vi "specu1a 1.0.0 Find Spectrometer by name.vi"(3 "All Spectrometers":T1[](array[typedef]) {"White"."Spectrum" format="%.2f"; "Data"."Spectrum" format="%.2f"; "Dark"."Spectrum" format="%.2f"}, 5 "Name":string) -> (0 "All Spectrometers out":T1[](array[typedef]) {"White"."Spectrum" format="%.2f"; "Data"."Spectrum" format="%.2f"; "Dark"."Spectrum" format="%.2f"}, 1 "Single Spectrometer":T1={"USB"={"pUSB"=0, "Pipe"=0, "No of Avgs"=0, "SYS Number"="", "DLL Number"=""}, "Unit Information"={"UnitID"="", "Sensor Name"="", "Serial Number"="", "Reserved"="", "Wave Upper"=630, "Wave Lower"=1050}, "Dark"={"Spectrum"=[], "Parameters"={"Integration time"=0, "Gain"=enum."Low", "TriggerEdge"=enum."Rising", "Trigger Mode"=enum."Internal", "Reserved"=0}, "No of Avgs"=0}, "Data"={"Spectrum"=[], "Parameters"={"Integration time"=0, "Gain"=enum."Low", "TriggerEdge"=enum."Rising", "Trigger Mode"=enum."Internal", "Reserved"=0}, "No of Avgs"=0}, "White"={"Spectrum"=[], "Parameters"={"Integration time"=10000, "Gain"=enum."Low", "TriggerEdge"=enum."Rising", "Trigger Mode"=enum."Internal", "Reserved"=0}, "No of Avgs"=0}, "Parameters"={"Integration time"=10000, "Gain"=enum."Low", "TriggerEdge"=enum."Rising", "Trigger Mode"=enum."Internal", "Reserved"=0}} {"White"."Spectrum" format="%.2f"; "Data"."Spectrum" format="%.2f"; "Dark"."Spectrum" format="%.2f"}, 2 "index of element":i32)   [LabVIEW 2010]
uses:
  Controls/specu1a 1.0.0 Single spectrometer.ctl
  Controls/specu1a 1.0.0 Product Information.ctl
  Controls/specu1a 1.0.0 Single measurement.ctl
  Controls/specu1a 1.0.0 Parameters.ctl
  Controls/specu1a 1.0.0 Trigger Edge.ctl
  Controls/specu1a 1.0.0 Trigger Mode.ctl
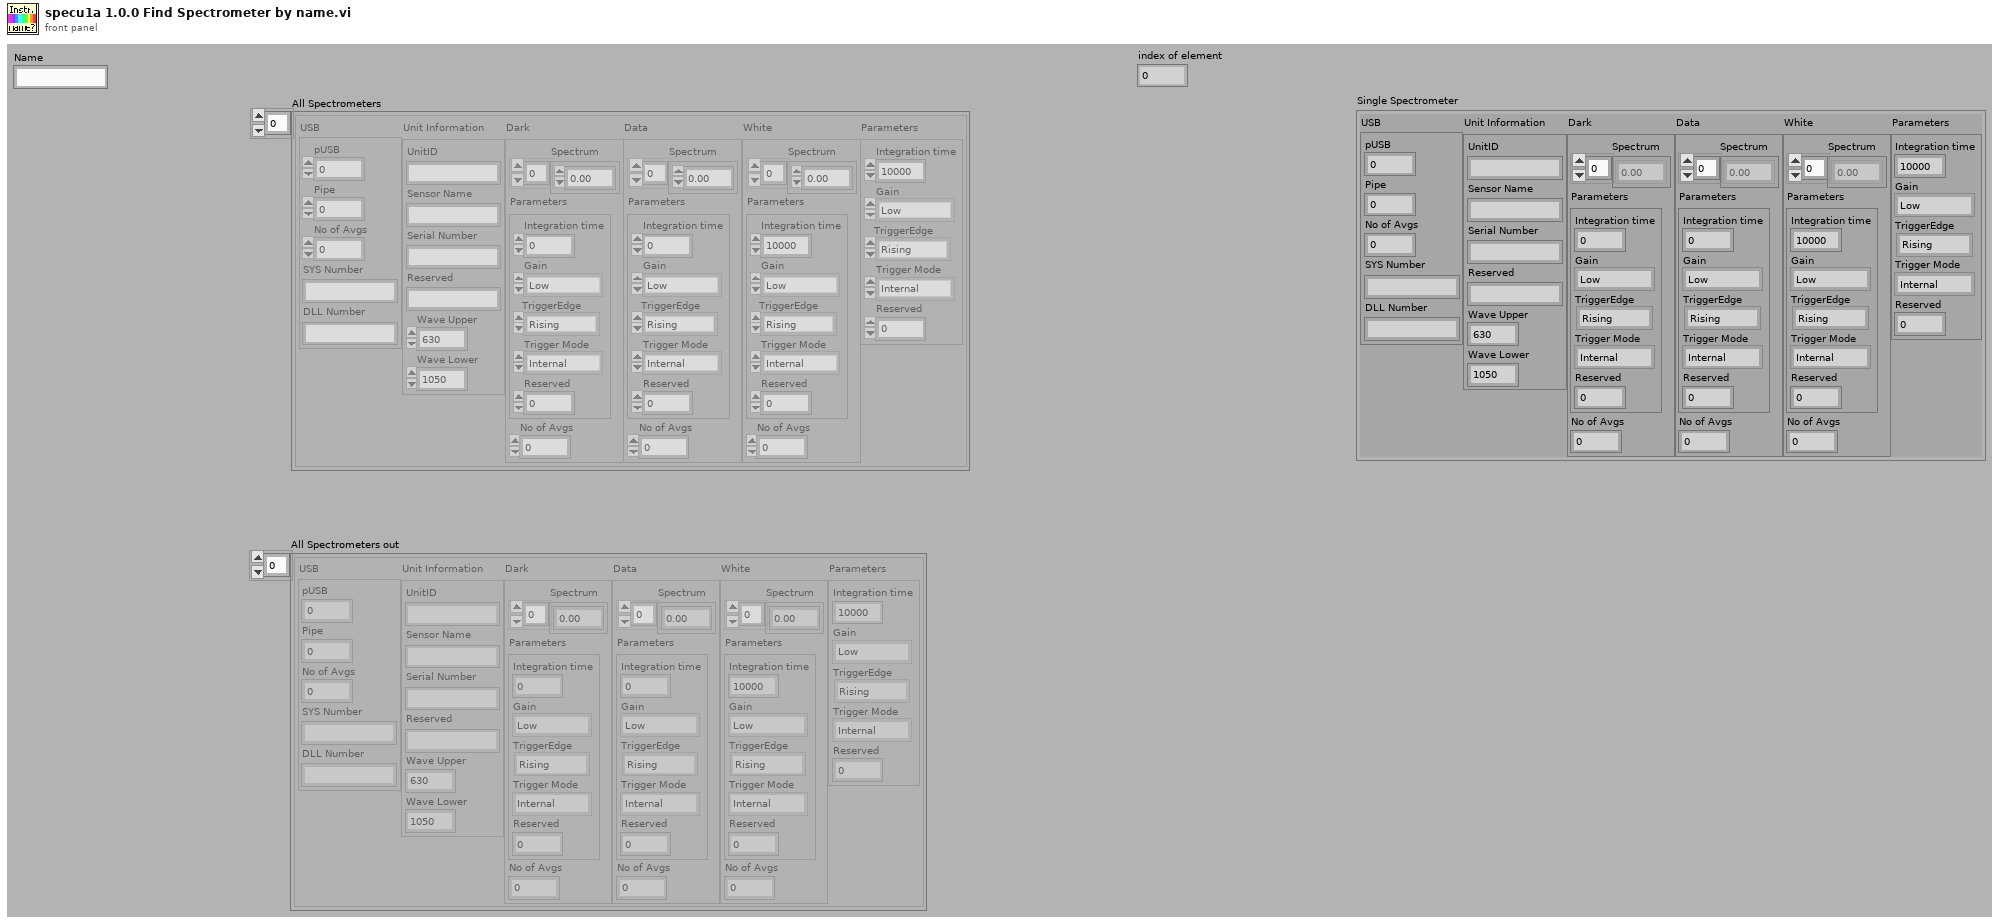
[diagram p1: front panel]
types:
  T1 = typedef "specu1a 1.0.0 Single spectrometer.ctl" = cluster{"USB":cluster{"pUSB":i32, "Pipe":i32, "No of Avgs":u32, "SYS Number":string, "DLL Number":string}, "Unit Information":T2, "Dark":T3, "Data":T3, "White":T3, "Parameters":T4}
  T2 = typedef "specu1a 1.0.0 Product Information.ctl" = cluster{"UnitID":string, "Sensor Name":string, "Serial Number":string, "Reserved":string, "Wave Upper":u16, "Wave Lower":u16}
  T3 = typedef "specu1a 1.0.0 Single measurement.ctl" = cluster{"Spectrum":dbl[], "Parameters":T4, "No of Avgs":u32}
  T4 = typedef "specu1a 1.0.0 Parameters.ctl" = cluster{"Integration time":u32, "Gain":enum16{"Low", "High", "No Function"}, "TriggerEdge":T5, "Trigger Mode":T6, "Reserved":u8}
  T5 = typedef "specu1a 1.0.0 Trigger Edge.ctl" = enum16{"Rising", "Falling", "No Function"}
  T6 = typedef "specu1a 1.0.0 Trigger Mode.ctl" = enum16{"Internal", "Asynchronous", "Synchronous"}
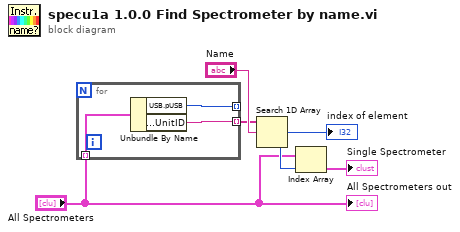
[diagram p0: block diagram]
diagram:
  n1 = for {
    tunnel: "All Spectrometers" -> [w8] mode=indexing
    tunnel: [w7] -> w2 mode=indexing
    tunnel: [w6] -> _ mode=indexing
    n2 = Unbundle By Name(w8) -> ("USB.pUSB"=w6:i32, "Unit Information.UnitID"=w7:string)
  }
  n3 = Search 1D Array(1D array=w2, element="Name") -> (index of element=w4:i32)  [unwired: 1 in]
  "index of element" <- w4
  n4 = Index Array(array="All Spectrometers", index=w4) -> (element=→"Single Spectrometer":T1)
  "All Spectrometers out" <- "All Spectrometers"
